vi "Write VAR.vi"(5 "Flow Meter DevID":i32=1, 7 "Timeout (ms)":u32, 8 "error in":errorcluster, 9 "Write Buffer":string, 10 "Variable to Write":T1, 11 "VISA resource name":refnum<visa-resource-name>) -> (0 "error out":errorcluster, 3 "VISA resource name out":refnum<visa-resource-name>)   [LabVIEW 2010, in "FEM-03.lvlib"]
uses:
  FEM-03.lvlib
  Private/Controls/Variable List.ctl
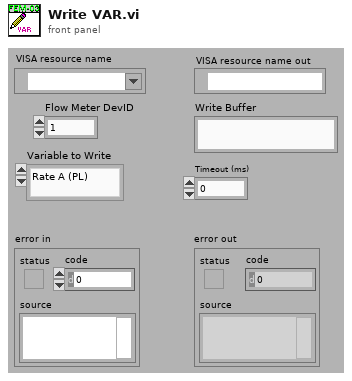
[diagram p1: front panel]
types:
  T1 = typedef "FEM-03.lvlib/Variable List.ctl" = enum16{"Rate A (PL)", "Rate A (GT)", "Job Total A", "Grand Total A", "A-KFR for Rate", "A-KFR decimal point location", "A-KFT for Total", "A-KFT decimal point location ", "A-Rate Engineering Units", "A-Total Engineering units", "A-Flow Direction", "Rate B (PL)", "Rate B (GT)", "Job Total B", "Grand Total B", "B-KFR for Rate", "B-KFR deciminal point location", "B-Rate Engineering units", "B-KFT for Total", "B-KFT decimal point location", "B-Total Engineering units", "Limit 1 Mode", "Limit1", "Margin 1 for rate limit", "Limit 2 Mode", "Limit2", "Margin 2 for rate limit", "Milli-amps Offset", "Milli-amps Out", "Analog Out Mode", "Serial Speed", "Unit Number", "Serial RESET TOTAL", "Update EEPROM", "Relay Override", "FORCE mA Output"}
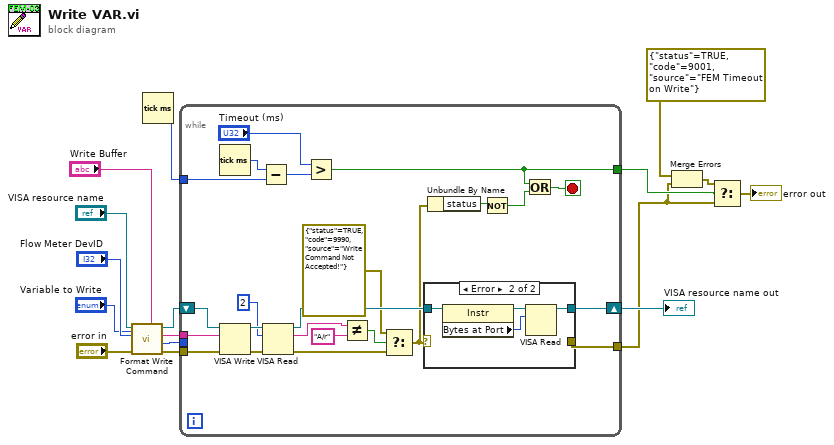
[diagram p0: block diagram]
diagram:
  n1 = call "Format Write Command.vi"("Write Buffer"="Write Buffer", "Variable to Read"="Variable to Write", "error in"="error in", "Flow Meter DevID"="Flow Meter DevID", "VISA resource name"="VISA resource name") -> ("error out"=w15:errorcluster, "Length Bytes (Dec)"=w10:i32, "Command String with Checksum"=w13:string, "VISA resource name out"=w14:refnum<visa-resource-name>)  [unwired: 3 in]
  n2 = Tick Count (ms)() -> (millisecond timer value=w8:u32)
  n3 = while {
    tunnel: w15 -> [w39]
    tunnel: w13 -> [w37]
    tunnel: w10 -> [_]
    shift-right: [w33] -> w9
    shift-left: w14 -> [w38]
    tunnel: [w32] -> w2
    tunnel: w8 -> [w30]
    tunnel: [w17] -> w3
    stop <- w18 stop-if-true
    n4 = Tick Count (ms)() -> (millisecond timer value=w31:u32)
    n5 = VISA Write(VISA resource name=w38, write buffer=w37, error in (no error)=w39) -> (VISA resource name out=w36:refnum<visa-resource-name>, error out=w35:errorcluster)  [unwired: 1 out]
    n6 = Subtract(x=w31, y=w30) -> (x-y=w28:u32)
    n7 = VISA Read(VISA resource name=w36, byte count=u32 2, error in (no error)=w35) -> (VISA resource name out=w34:refnum<visa-resource-name>, read buffer=w26:string, error out=w23:errorcluster)  [unwired: 1 out]
    n8 = Greater?(x="Timeout (ms)", y=w28) -> (0:w17:bool)
    n9 = Not Equal?(x=w26, y="A/r") -> (x != y?=w24:bool)
    n10 = Select(t=errorcluster {"status"=TRUE, "code"=9990, "source"="Write Command Not Accepted!"}, s=w24, f=w23) -> (s? t:f=w21:errorcluster)
    n11 = case shown="Error" w21 {
      selector: w21 -> [w41 _]
      tunnel: w34 -> [w40 w45]
      tunnel: [w40 w42] -> w33
      tunnel: [w41 _] -> w32
      frame No Error {
      }
      frame Error {
        n12 = property class="Instr"(reference=w45) -> (reference out=w44:refnum<visa-resource-name>, "Bytes at Port"=w43:u32)  [unwired: 1 in, 1 out]
        n13 = VISA Read(VISA resource name=w44, byte count=w43) -> (VISA resource name out=w42:refnum<visa-resource-name>)  [unwired: 1 in, 3 out]
      }
    }
    n14 = Unbundle By Name(w21) -> ("status"=w20:bool)
    n15 = Not(x=w20) -> (.not. x?=w19:bool)
    n16 = Or(x=w17, y=w19) -> (x .or. y?=w18:bool)
  }
  "VISA resource name out" <- w9
  n17 = Merge Errors(errorcluster {"status"=TRUE, "code"=9001, "source"="FEM Timeout on Write"} ("error out"), w2) -> (w4:errorcluster)
  n18 = Select(t=w4, s=w3, f=w2) -> (s? t:f=→"error out":errorcluster)
